vi "openRS232.vi"(0 "com":refnum<visa-resource-name>="COM1") -> (1 "VISA resource name":refnum<visa-resource-name>, 2 "error out":errorcluster)   [LabVIEW 2011]
uses:
  <vilib>/Instr/_visa.llb/VISA Configure Serial Port (Instr).vi
panel:
  in  "baud rate (115200":u32=115200
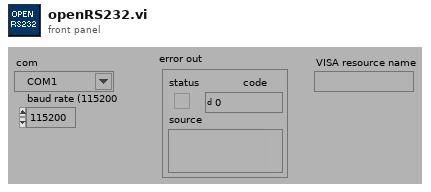
[diagram p1: front panel]
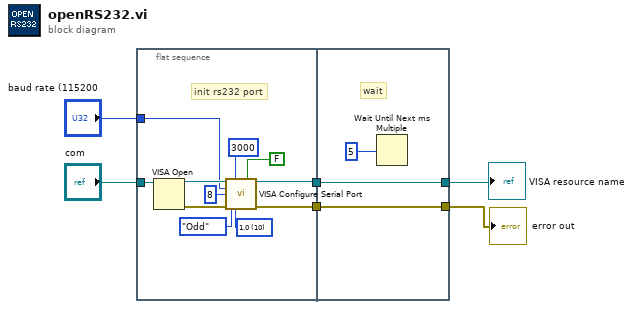
[diagram p0: block diagram]
diagram:
  n1 = flat-sequence {
    tunnel: "com" -> [w10]
    tunnel: "baud rate (115200" -> [w9]
    tunnel: [w8] -> w4
    tunnel: [w7] -> w1
    tunnel: w4 -> [w19]
    tunnel: [w19] -> w3
    tunnel: [w18] -> w2
    tunnel: w1 -> [w18]
    frame #0 {
      w14 = u16 10 items=["1.0"=10, "1.5"=15, "2.0"=20] ("stop bits (10: 1 bit)")
      # "init rs232 port"
      n2 = VISA Open(VISA resource name=w10) -> (VISA resource name=w16:refnum<visa-resource-name>, error out=w15:errorcluster)  [unwired: 4 in]
      n3 = call-poly "VISA Configure Serial Port"("VISA resource name"=w16, "timeout (10sec)"=u32 3000, "Enable Termination\nChar (T)"=FALSE ("Enable Termination\nChar (T)"), "baud rate (9600)"=w9, "data bits (8)"=u16 8, "parity (0:none)"=enum16{"None", "Odd", "Even", "Mark", "Space"}."Odd", "error in (no error)"=w15, "stop bits (10: 1 bit)"=w14) -> ("VISA resource name out"=w8:refnum<visa-resource-name>, "error out"=w7:errorcluster)  [unwired: 6 in]
    }
    frame #1 {
      # "wait"
      n4 = Wait Until Next ms Multiple(millisecond multiple=u32 5 ("millisecond timer value")) -> ()  [unwired: 1 out]
    }
  }
  "error out" <- w2
  "VISA resource name" <- w3
